vi "Launcher.vi"() -> ()   [LabVIEW 2020]
uses:
  <vilib>/ActorFramework/Message Enqueuer/Message Enqueuer.lvclass
  Business Logic/Business Logic/Business Logic.lvclass
  C:/Program Files (x86)/National Instruments/LabVIEW 2020/vi.lib/ActorFramework/Actor/Actor.lvclass
  Business Logic/Business Logic/Business Logic.lvclass/Business Logic.ctl
  <vilib>/ActorFramework/Message Enqueuer/Message Enqueuer.lvclass/Message Enqueuer.ctl
  Business Logic/Business Logic/Write HW ID.vi
  <vilib>/ActorFramework/Message Enqueuer/Enqueue.vi
  <vilib>/ActorFramework/Stop Msg/Stop Msg.lvclass
  C:/Program Files (x86)/National Instruments/LabVIEW 2020/vi.lib/ActorFramework/Message/Message.lvclass
  <vilib>/ActorFramework/Message Priority Queue/Priority Enqueue.vi
  <vilib>/ActorFramework/Actor/Actor.lvclass
panel:
  in  "New":bool
  in  "stop":bool
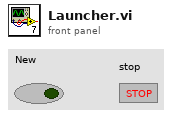
[diagram p1: front panel]
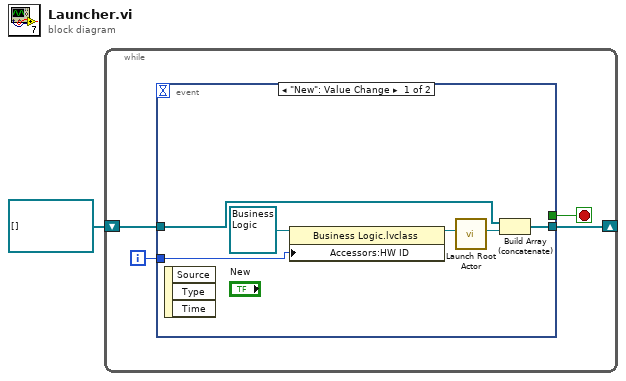
[diagram p0: block diagram]
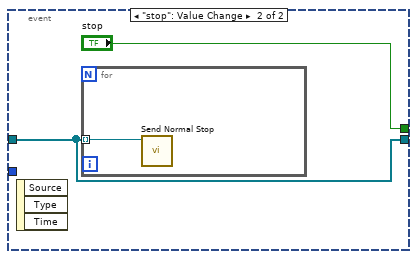
[diagram p2: hidden frame]
diagram:
  n1 = while {
    shift-right: [w5] -> _
    shift-left: refnum<class "Message Enqueuer.lvclass">[] [] -> [w4]
    i -> [w2]
    stop <- w3 stop-if-true
    n2 = event shown="[0] \"New\": Value Change" {
      selector: _ -> [_ _]
      dyn-events: _ -> [_ _]
      timeout: _ -> [_ _]
      tunnel: [w11 w12] -> w5
      tunnel: w4 -> [w10 w12]
      tunnel: [_ "stop"] -> w3
      tunnel: w2 -> [w6 _]
      event "New": Value Change {
        n3 = event-data() -> ()  [unwired: 1 in, 3 out]
        n4 = property class="Business Logic.lvclass"(reference=refnum<class "Business Logic.lvclass"> refnum ("Business Logic.lvlib:Business Logic.lvclass"), "Accessors:HW ID"=w6) -> (reference out=w7:refnum<class "Business Logic.lvclass">)  [unwired: 1 in, 1 out]
        n5 = call <vilib>:"Launch Root Actor.vi"("Actor"=w7) -> ("Actor's Enqueuer"=w8:refnum<class "Message Enqueuer.lvclass">)  [unwired: 9 in, 1 out]
        n6 = Build Array (concatenate)(w10, w8) -> (w11:refnum<class "Message Enqueuer.lvclass">[])
      }
      event "stop": Value Change {
        n7 = event-data() -> ()  [unwired: 1 in, 3 out]
        n8 = for {
          tunnel: w12 -> [w14] mode=indexing
          n9 = call <vilib>:"Send Normal Stop.vi"("Message Enqueuer"=w14) -> ()  [unwired: 10 in, 1 out]
        }
      }
    }
  }
